vi "FUG-HCN.contents.vi"   [LabVIEW 2014, in "FUG-HCN.lvlib"]
doc: "The class is communicating with PROBUS device, which controls the HV power supply of the CAGE."
uses:
  FUG-HCN.lvlib
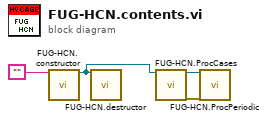
[diagram p0: block diagram]
diagram:
  n1 = call "FUG-HCN.constructor.vi"("name"="") -> ("i ref out"=w1:refnum<vi>)  [unwired: 16 in, 2 out]
  n2 = call "FUG-HCN.destructor.vi"("i ref in"=w1) -> ()  [unwired: 18 in, 1 out]
  n3 = call "FUG-HCN.ProcCases.vi"("i ref in"=w1) -> ("i ref out"=w4:refnum<vi>, "error out"=w3:errorcluster)  [unwired: 16 in, 1 out]
  n4 = call "FUG-HCN.ProcPeriodic.vi"("i ref in"=w4, "error in (no error)"=w3) -> ()  [unwired: 15 in, 3 out]
